vi "KE622x -- DCon Mode Get Params.vi"(0 "Resource In":refnum<visa-resource-name>, 1 "Check For SCPI Errors? (T)":bool=TRUE, 11 "error in (no error)":errorcluster) -> (4 "Resource Out (dupl)":refnum<visa-resource-name>, 8 "Differential Cond Params":T1={"Start Value (A)"=0.0, "Stop Value (A)"=-1e-05, "Step Size (A)"=1e-05, "Delta Value (A)"=1e-06, "Delay (s)"=1e-06, "Abort On\nCompliance?"=FALSE} {"Delay (s)" min=0.001 max=9999.999 format="%.3f"; "Delta Value (A)" min=0.0 max=0.105 format="%.3p"; "Step Size (A)" min=0.0 max=0.105 format="%.3p"; "Stop Value (A)" min=-0.105 max=0.105 format="%.3p"; "Start Value (A)" min=-0.105 max=0.105 format="%.3p"}, 15 "error out":errorcluster)   [LabVIEW 2019, in "Keithley 622x.lvlib"]
doc: "Returns the parameters for 'Differntial Conductance' measurements. Note that performing this measurement implies that the 622x is being used in conjuction with a 2182/2182A nano-voltmeter."
uses:
  Keithley 622x.lvlib
  Typedefs/KE622x -- DCon Mode Params.ctl
  Low Level/Typedefs/KE622x -- DCon Mode Start Stop Level.ctl
  Low Level/Typedefs/KE622x -- DCon Mode Step Delta Size.ctl
  Low Level/Typedefs/KE622x -- Delta DCon Mode Delay.ctl
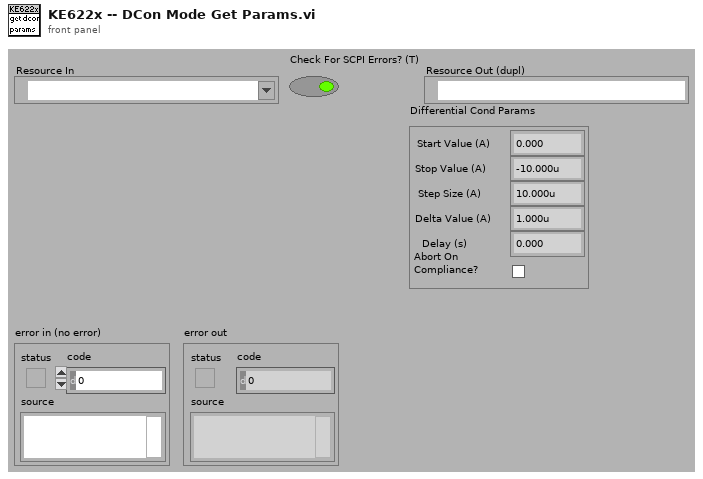
[diagram p1: front panel]
types:
  T1 = typedef "Keithley 622x.lvlib/KE622x -- DCon Mode Params.ctl" = cluster{"Start Value (A)":T2, "Stop Value (A)":T2, "Step Size (A)":T3, "Delta Value (A)":T3, "Delay (s)":T4, "Abort On\nCompliance?":bool}
  T2 = typedef "Keithley 622x.lvlib/KE622x -- DCon Mode Start Stop Level.ctl" = dbl
  T3 = typedef "Keithley 622x.lvlib/KE622x -- DCon Mode Step Delta Size.ctl" = dbl
  T4 = typedef "Keithley 622x.lvlib/KE622x -- Delta DCon Mode Delay.ctl" = dbl
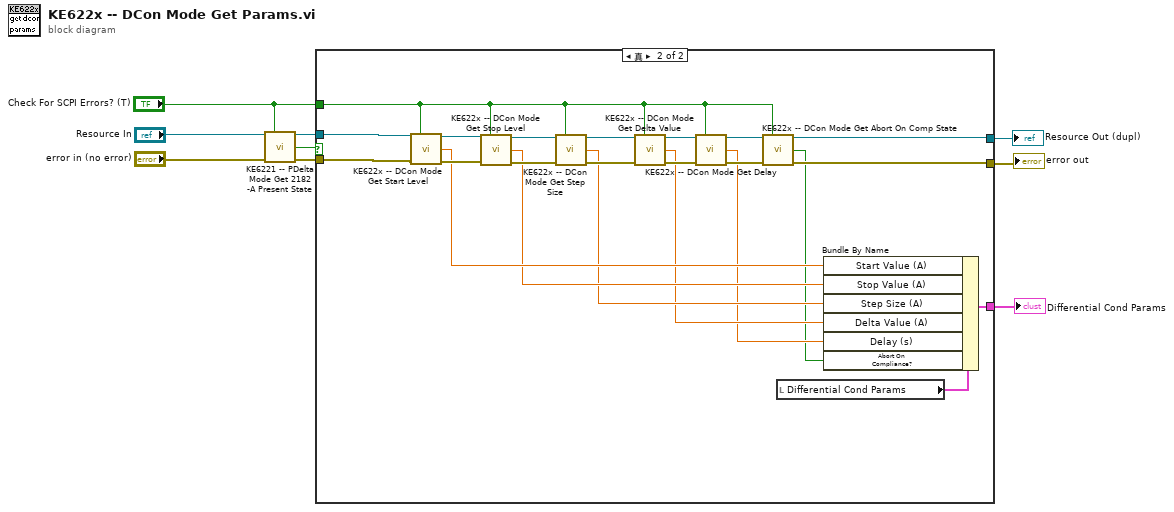
[diagram p0: block diagram]
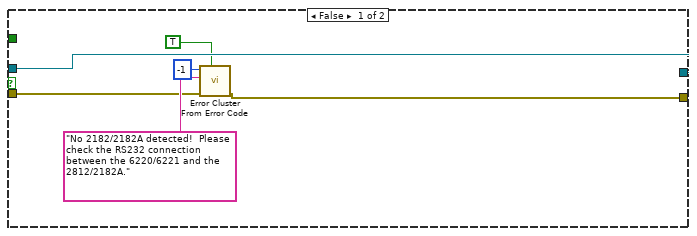
[diagram p2: hidden frame]
diagram:
  n1 = call "KE6221 -- PDelta Mode Get 2182 -A Present State.vi"("Resource In"="Resource In", "Check For SCPI Errors? (T)"="Check For SCPI Errors? (T)", "error in (no error)"="error in (no error)") -> ("Resource Out (dupl)"=w9:refnum<visa-resource-name>, "2182/2182A Present?"=w2:bool, "error out"=w8:errorcluster)  [unwired: 10 in]
  n2 = case shown="真" w2 {
    tunnel: [_ w24] -> w1
    tunnel: w9 -> [w12 w17]
    tunnel: w8 -> [w13 w16]
    tunnel: "Check For SCPI Errors? (T)" -> [_ w23]
    tunnel: [w12 w22] -> w4
    tunnel: [w11 w21] -> w3
    frame False {
      n3 = call <vilib>:"Error Cluster From Error Code.vi"("show call chain? (False)"=TRUE, "error in (no error)"=w13, "error message (\"\")"="No 2182/2182A detected!  Please check the RS232 connection between the 6220/6221 and the 2812/2182A.", "error code (0)"=-1) -> ("error out"=w11:errorcluster)  [unwired: 5 in]
    }
    frame True {
      n4 = call "KE622x -- DCon Mode Get Start Level.vi"("Resource In"=w17, "Check For SCPI Errors? (T)"=w23, "error in (no error)"=w16) -> ("Resource Out (dupl)"=w38:refnum<visa-resource-name>, "Start Level (A)"=w27:T2, "error out"=w37:errorcluster)  [unwired: 10 in]
      n5 = call "KE622x -- DCon Mode Get Stop Level.vi"("Resource In"=w38, "Check For SCPI Errors? (T)"=w23, "error in (no error)"=w37) -> ("Resource Out (dupl)"=w36:refnum<visa-resource-name>, "Stop Level (A)"=w26:T2, "error out"=w35:errorcluster)  [unwired: 10 in]
      n6 = call "KE622x -- DCon Mode Get Step Size.vi"("Resource In"=w36, "Check For SCPI Errors? (T)"=w23, "error in (no error)"=w35) -> ("Resource Out (dupl)"=w32:refnum<visa-resource-name>, "Step Size (A)"=w25:T3, "error out"=w31:errorcluster)  [unwired: 10 in]
      n7 = call "KE622x -- DCon Mode Get Delta Value.vi"("Resource In"=w32, "Check For SCPI Errors? (T)"=w23, "error in (no error)"=w31) -> ("Resource Out (dupl)"=w34:refnum<visa-resource-name>, "Delta Value (A)"=w20:T3, "error out"=w33:errorcluster)  [unwired: 10 in]
      n8 = call "KE622x -- DCon Mode Get Delay.vi"("Resource In"=w34, "Check For SCPI Errors? (T)"=w23, "error in (no error)"=w33) -> ("Resource Out (dupl)"=w30:refnum<visa-resource-name>, "Delay (s)"=w19:T4, "error out"=w29:errorcluster)  [unwired: 10 in]
      n9 = call "KE622x -- DCon Mode Get Abort On Comp State.vi"("Resource In"=w30, "Check For SCPI Errors? (T)"=w23, "error in (no error)"=w29) -> ("Resource Out (dupl)"=w22:refnum<visa-resource-name>, "Abort On Compliance?"=w18:bool, "error out"=w21:errorcluster)  [unwired: 10 in]
      n10 = local read "Differential Cond Params"() -> (w28:T1)
      n11 = Bundle By Name(cluster=w28, "Start Value (A)"=w27, "Stop Value (A)"=w26, "Step Size (A)"=w25, "Delta Value (A)"=w20, "Delay (s)"=w19, "Abort On\nCompliance?"=w18) -> (w24:T1)
    }
  }
  "Resource Out (dupl)" <- w4
  "error out" <- w3
  "Differential Cond Params" <- w1
